vi "_시리얼_Mark10-헤드이동.vi"(4 "동작 모드":string(combo)="STOP", 5 "시리얼 포트":refnum<visa-resource-name>="COM5") -> (2 "VISA 리소스 이름 출력":refnum<visa-resource-name>)   [LabVIEW 2015]
panel:
  # "MARK10 헤드 이동 제어"
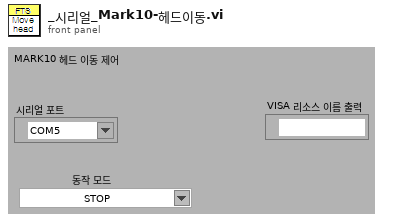
[diagram p1: front panel]
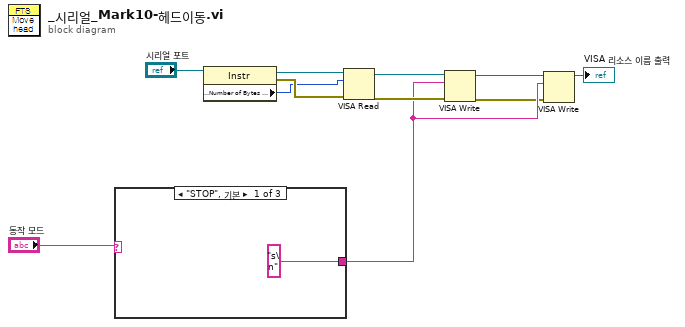
[diagram p0: block diagram]
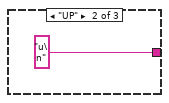
[diagram p2: hidden frame]
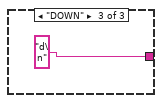
[diagram p3: hidden frame]
diagram:
  n1 = case shown="\"STOP\", 기본" "동작 모드" {
    tunnel: ["s\n" "u\n" "d\n"] -> w3
    frame "STOP", Default {
    }
    frame "UP" {
    }
    frame "DOWN" {
    }
  }
  n2 = property class="Instr"(reference="시리얼 포트") -> (reference out=w11:refnum<visa-resource-name>, error out=w9:errorcluster, "Serial Settings:Number of Bytes at Serial Port"=w6:u32)  [unwired: 1 in]
  n3 = VISA Read(VISA resource name=w11, byte count=w6, error in (no error)=w9) -> (VISA resource name out=w8:refnum<visa-resource-name>, error out=w7:errorcluster)  [unwired: 2 out]
  n4 = VISA Write(VISA resource name=w8, write buffer=w3, error in (no error)=w7) -> (VISA resource name out=w4:refnum<visa-resource-name>, error out=w2:errorcluster)  [unwired: 1 out]
  n5 = VISA Write(VISA resource name=w4, write buffer=w3, error in (no error)=w2) -> (VISA resource name out=→"VISA 리소스 이름 출력":refnum<visa-resource-name>)  [unwired: 2 out]
